vi "Read Warm-Up Time.vi"(8 "error in (no error)":errorcluster, 11 "Abstract Display in":refnum<class "Abstract Display.lvclass">) -> (0 "error out":errorcluster, 2 "Warm-Up Time":dbl, 3 "Abstract Display out":refnum<class "Abstract Display.lvclass">)   [LabVIEW 2013, in "Display Panel.lvlib" / "Abstract Display.lvclass"]
uses:
  Abstract Display.lvclass
  Abstract Display.lvclass/Abstract Display.ctl
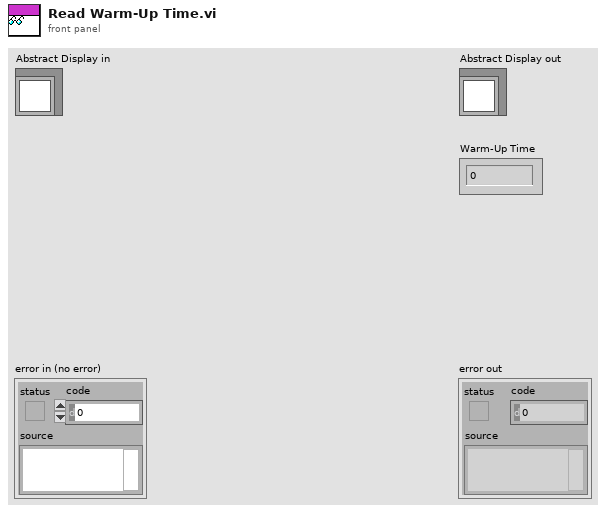
[diagram p1: front panel]
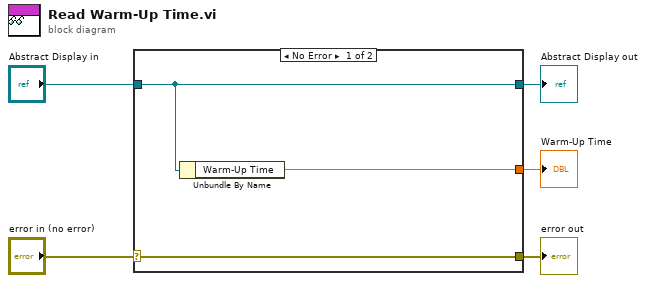
[diagram p0: block diagram]
diagram:
  n1 = case shown="No Error" "error in (no error)" {
    selector: "error in (no error)" -> [w8 w9]
    tunnel: [w8 w9] -> w4
    tunnel: [w7 w10] -> w2
    tunnel: "Abstract Display in" -> [w7 w10]
    tunnel: [w6 _] -> w1
    frame No Error {
      n2 = Unbundle By Name(w7) -> ("Warm-Up Time"=w6:dbl)
    }
    frame Error {
    }
  }
  "error out" <- w4
  "Abstract Display out" <- w2
  "Warm-Up Time" <- w1
